vi "qVEL.vi"(0 "System no.":i32=1 min=1 max=4 step=1, 2 "Axes to query":string[](array[string]), 3 "All axes?":bool, 4 "Axis identifier?":bool=TRUE, 5 "error in":errorcluster) -> (14 "Velocity":dbl[](array[numeric]) format="%.6f", 19 "error out":errorcluster)   [LabVIEW 2026]
doc: "Returns velocity setting for specified axes.\n\nAnalog: If All axes? = TRUE, then Axis identifier? can be FALSE; Velocity unit is µm/s\n\nC-702, C-848, Mercury: If All axes? = TRUE, then Axis identifier? can be FALSE\n\nC-843, C-843.PM, C-844, E-516: If All axes? = TRUE, then Axis identifier? must be TRUE\n\nC-413, C-865, C-866, C-867, C-877, C-884, C-891, Hydra, Pollux, Mercury_GCS: If All axes? = TRUE, then Axis identifier? can be FALSE. Velocity unit is mm/s.\n\nC-880: If All axes? = TRUE, then Axis identifier? can be FALSE. NanoCube axes will report velocity = 0\n\nC-880K005: VI only supported when called through PI_Multix.vi\n\nC-885: If All axes? = TRUE, then Axis identifier? can be FALSE.\n\nC-886: If All axes? = TRUE, then Axis identifier? can be FALSE. VEL? only reports the velocity for additional axes. To query the velocity of the parallel kinematics (system velocity), please use the VLS? command instead.\n\nE-517, E-518: If All axes? = TRUE, then Axis identifier? can be FALSE. Velocity unit is µm/s in closed-loop operation and V/s in open-loop operation.\n\nE-710: If All axes? = TRUE, then Axis identifier? must be TRUE. Velocity unit is µm/ms.\n\nE-709, E-712, E-725, E-727, E-753, E-754, E-861: If All axes? = TRUE, then Axis identifier? can be FALSE. Velocity unit is µm/s. \n\nE-755: If All axes? = TRUE, then Axis identifier? can be FALSE. Velocity unit is µm/s. Command not available for E-755.101.\n\nE-761: If All axes? = TRUE, then Axis identifier? can be FALSE. Velocity unit is µm/ms.\n\nC-887, F-206, M-8X0: For GCS syntax version = GCS 2.0 or higher (check with CSV?.vi. If CSV?.vi is not supported, syntax version is GCS 1.0), only valid for velocity of axes A and/or B. All axes? must be FALSE. For platform velocity, use VLS? instead. For axes K,L,M command is not valid.\nFor GCS syntax version = GCS 1.0, Velocity of platform: All axes? = TRUE AND Axis identifier? = FALSE; velocity of axes A,B: All axes? must be FALSE; axes K,L,M: command not valid. For platform velocity: only first field of velocity array is valid\n\nE-873, E-874: If All axes? = TRUE, then Axis identifier? can be FALSE."
uses:
  Controller names.ctl
  Communication/Syntax.ctl
  Communication/Global1.vi
  Global2 (Array).vi
panel:
  # "Returns velocity setting for specified axes."
  # "If all axes: use"
  # "Query"
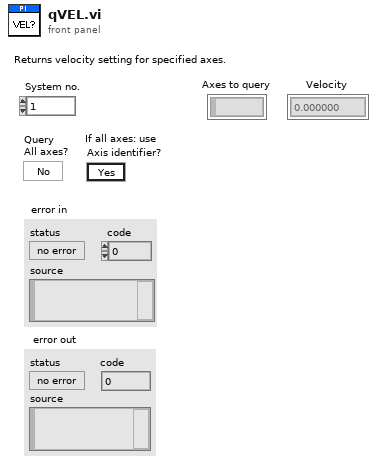
[diagram p1: front panel]
types:
  T1 = typedef "Syntax.ctl" = enum16{"GCS 1.0", "GCS 2.0", "GCS 3.0"}
  T2 = typedef "Controller names.ctl" = enum16{"None", "Analog", "C-702", "C-413", "C-414", "C-843", "C-843.PM", "C-844", "C-848", "C-865", "C-866", "C-867", "C-877", "C-880", "C-884", "C-885", "C-886", "C-887", "C-891", "E-135", "E-516", "E-517", "E-518", "E-709", "E-710", "E-712", "E-725", "E-727", "E-753", "E-754", "E-755", "E-761", "E-816", "E-861", "E-870", "E-871", "E-872", "E-873", "E-874", "F-206", "HydraPollux", "M-840", "M-850", "M-8X0", "Mercury", "Mercury_GCS", "PI_GCS2"}
  T3 = cluster{"Conn. axes":string[], "Controller name":T2}[]
  T4 = cluster{"Conn. axes":string[], "Controller name":T2}
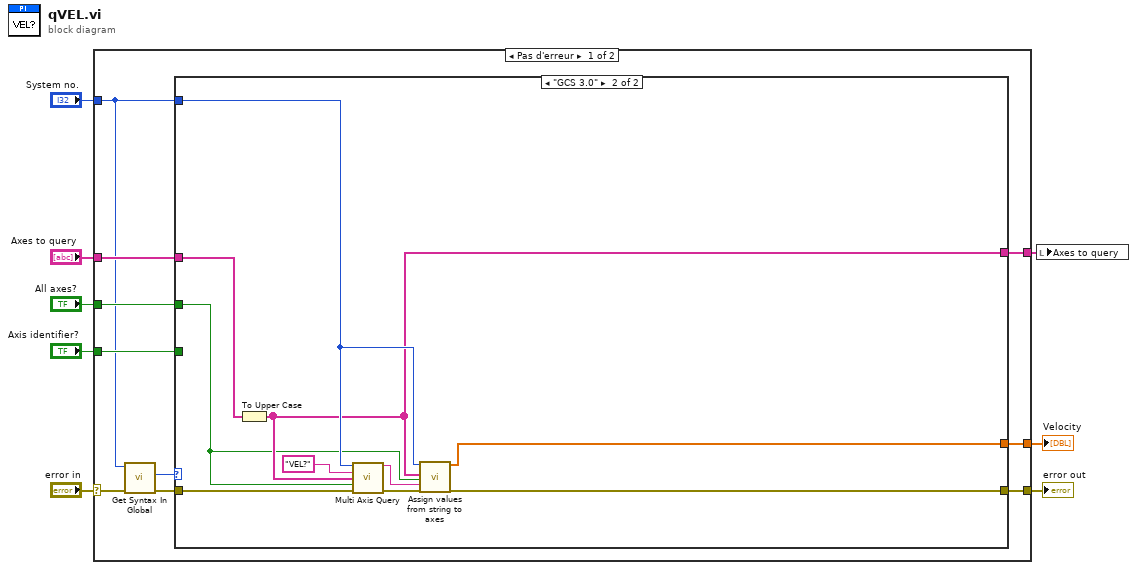
[diagram p0: block diagram]
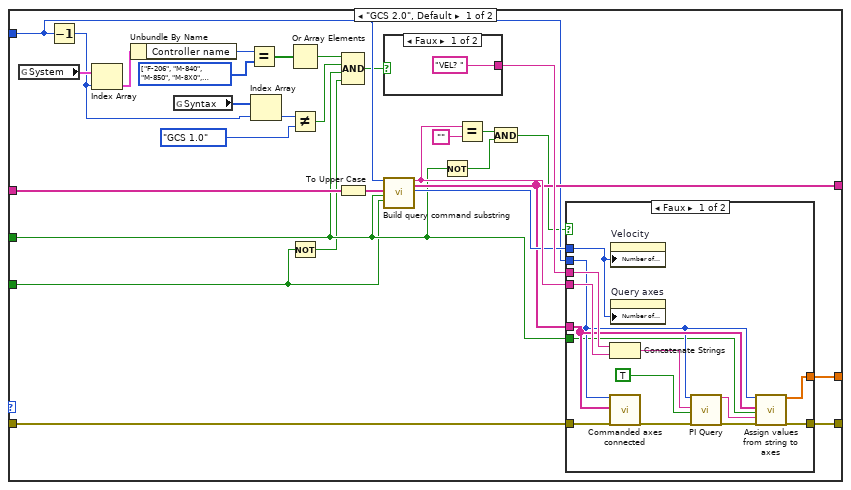
[diagram p2: hidden frame]
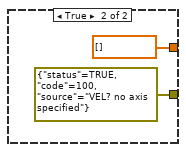
[diagram p3: hidden frame]
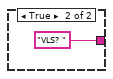
[diagram p4: hidden frame]
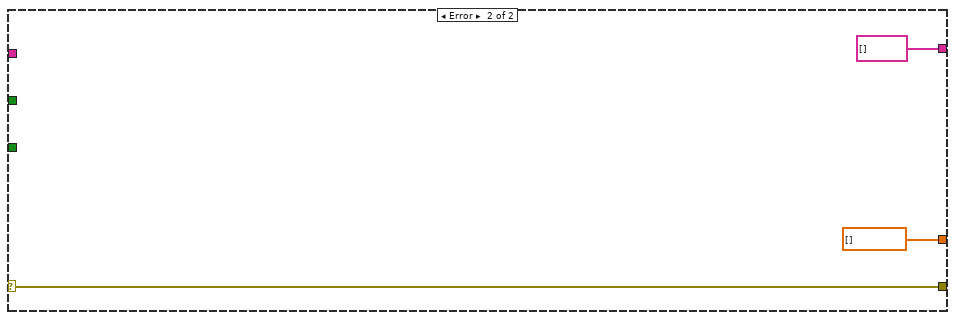
[diagram p5: hidden frame]
diagram:
  n1 = case shown="Pas d'erreur" "error in" {
    selector: "error in" -> [w11 w76]
    tunnel: [w18 dbl[] [] ("Values")] -> w8
    tunnel: "Axes to query" -> [w17 _]
    tunnel: [w13 w76] -> w6
    tunnel: "Axis identifier?" -> [w14 _]
    tunnel: "System no." -> [w9 _]
    tunnel: [w16 string[] [] ("Axes to query out")] -> w3
    tunnel: "All axes?" -> [w15 _]
    frame No Error {
      n2 = call "Get Syntax In Global.vi"("error in"=w11, "System no."=w9) -> ("error out"=w10:errorcluster, "Syntax"=w12:T1)  [unwired: 8 in]
      n3 = case shown="\"GCS 3.0\"" w12 {
        tunnel: [w46 w68] -> w18
        tunnel: w17 -> [w45 w72]
        tunnel: [w40 w67] -> w16
        tunnel: w9 -> [w33 w71]
        tunnel: w15 -> [w25 w66]
        tunnel: w14 -> [w24 _]
        tunnel: w10 -> [w22 w70]
        tunnel: [w21 w69] -> w13
        frame "GCS 2.0", Default {
          w30 = T2[] [enum."F-206", enum."M-840", enum."M-850", enum."M-8X0", enum."C-887"] items=["None", "Analog", "C-702", "C-413", "C-414", "C-843", "C-843.PM", "C-844", "C-848", "C-865", "C-866", "C-867", "C-877", "C-880", "C-884", "C-885", "C-886", "C-887", "C-891", "E-135", "E-516", "E-517", "E-518", "E-709", "E-710", "E-712", "E-725", "E-727", "E-753", "E-754", "E-755", "E-761", "E-816", "E-861", "E-870", "E-871", "E-872", "E-873", "E-874", "F-206", "HydraPollux", "M-840", "M-850", "M-8X0", "Mercury", "Mercury_GCS", "PI_GCS2"]
          n4 = global read "Global2 (Array).vi" "System"() -> (w35:T3)
          n5 = Decrement(x=w33) -> (x-1=w34:i32)
          n6 = Index Array(array=w35, index=w34) -> (element=w32:T4)
          n7 = Unbundle By Name(w32) -> ("Controller name"=w31:T2)
          n8 = global read "Global1.vi" "Syntax"() -> (w37:T1[])
          n9 = Equal?(x=w31, y=w30) -> (x = y?=w29:bool[])
          n10 = Index Array(array=w37, index=w34) -> (element=w36:T1)
          n11 = Or Array Elements(Boolean array=w29) -> (logical OR=w28:bool)
          n12 = Not Equal?(x=w36, y=Syntax."GCS 1.0" ("element")) -> (x != y?=w27:bool)
          n13 = Not(x=w24) -> (.not. x?=w23:bool)
          n14 = To Upper Case(1:w45) -> (0:w43:string[])
          n15 = Compound Arithmetic op=AND(w28, w27, w25, w23) -> (w26:bool)
          n16 = case shown="Faux" w26 {
            tunnel: ["VEL? " "VLS? "] -> w47
            frame False {
            }
            frame True {
            }
          }
          n17 = call "Build query command substring.vi"("System no."=w33, "Axes to query in"=w43, "Query\nAll axes?"=w25, "For all axes: use\nAxis identifier?"=w24) -> ("Command substring"=w42:string, "Axes to query out"=w40:string[], "Number of rows"=w41:u32)  [unwired: 2 in, 11 out]
          n18 = Not(x=w25) -> (.not. x?=w38:bool)
          n19 = Equal?(x=w42, y="" ("x")) -> (x = y?=w39:bool)
          n20 = And(x=w39, y=w38) -> (x .and. y?=w20:bool)
          n21 = case shown="Faux" w20 {
            tunnel: w47 -> [w60 _]
            tunnel: [w58 dbl[] [] ("Values")] -> w46
            tunnel: w42 -> [w57 _]
            tunnel: w41 -> [w56 _]
            tunnel: w40 -> [w55 _]
            tunnel: w33 -> [w53 _]
            tunnel: w25 -> [w52 _]
            tunnel: w22 -> [w51 _]
            tunnel: [w48 errorcluster {"status"=TRUE, "code"=100, "source"="VEL? no axis specified"} ("error out")] -> w21
            frame False {
              n22 = Concatenate Strings(w60, w57) -> (w59:string)
              n23 = call "Commanded axes connected.vi"("System no."=w53, "Commanded axes"=w55, "error in"=w51) -> ("error out"=w54:errorcluster)  [unwired: 1 in, 15 out]
              n24 = property on="Velocity" class="Tabl (strict)"("Number of Rows"=w56) -> ()  [unwired: 2 in, 2 out]
              n25 = property on="Query axes" class="Tabl (strict)"("Number of Rows"=w56) -> ()  [unwired: 2 in, 2 out]
              n26 = call "PI Query.vi"("System no."=w53, "String to send"=w59, "Attach termination char.?"=TRUE ("Attach Linefeed?"), "error in"=w54) -> ("String read"=w49:string, "error out"=w50:errorcluster)  [unwired: 3 in, 11 out]
              n27 = call "Assign values from string to axes.vi"("System no."=w53, "Queried axes"=w55, "All axes queried?"=w52, "Input String"=w49, "error in"=w50) -> ("Values"=w58:dbl[], "error out"=w48:errorcluster)  [unwired: 4 in, 9 out]
            }
            frame True {
            }
          }
        }
        frame "GCS 3.0" {
          n28 = To Upper Case(1:w72) -> (0:w67:string[])
          n29 = call "Multi Axis Query.vi"("System no."=w71, "Command"="VEL?", "Axis"=w67, "All axes?"=w66, "error in (no error)"=w70) -> ("Answer"=w73:string, "error out"=w74:errorcluster)  [unwired: 9 in]
          n30 = call "Assign values from string to axes.vi"("System no."=w71, "Queried axes"=w67, "All axes queried?"=w66, "Input String"=w73, "error in"=w74) -> ("Values"=w68:dbl[], "error out"=w69:errorcluster)  [unwired: 4 in, 9 out]
        }
      }
    }
    frame Error {
    }
  }
  "error out" <- w6
  "Velocity" <- w8
  n31 = local write "Axes to query"(w3) -> ()
